vi "Pneumatic Sucker Relax.vi"(8 "error in":errorcluster, 10 "relax sec":dbl=0.2 format="%#_13g") -> (0 "error out":errorcluster)   [LabVIEW 2019]
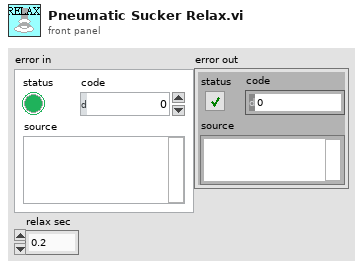
[diagram p1: front panel]
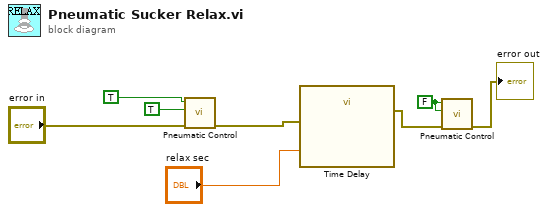
[diagram p0: block diagram]
diagram:
  w3 = FALSE ("ENA")
  n1 = call "Pneumatic Control.vi"("error in"="error in", "DIR"=TRUE, "ENA"=TRUE) -> ("error out"=w6:errorcluster)  [unwired: 8 in]
  n2 = call "Time Delay"("error in (no error)"=w6, "Delay Time (s)"="relax sec") -> ("error out"=w4:errorcluster)  [unwired: 9 in]
  n3 = call "Pneumatic Control.vi"("error in"=w4, "DIR"=w3, "ENA"=w3) -> ("error out"=→"error out":errorcluster)  [unwired: 8 in]
